vi "KE6221 -- Get Arb Wave Params.vi"(0 "Resource In":refnum<visa-resource-name>, 1 "Check For SCPI Errors? (T)":bool=TRUE, 11 "error in (no error)":errorcluster, 13 "Timeout (10000 ms)":u32=10000) -> (4 "Resource Out (dupl)":refnum<visa-resource-name>, 8 "Arb Wave Params":T1={"Frequency (Hz)"=1000.0, "Amplitude (A)"=0.001, "Offset (A)"=0.0, "Ranging Mode"=enum."Best", "Fixed Range"=enum."2mA", "Playback Mode"=enum."Time", "Time (s)"=1.0, "Num Cycles"=1.0, "Phase\nMarker?"=FALSE, "Phase Marker (deg)"=180.0, "Trig Link Line"=enum."1", "Arb Waveform Points"=[], "Num Arb Points"=0} {"Arb Waveform Points" min=-1.0 max=1.0 format="%.3f"; "Offset (A)" min=-0.105 max=0.105 format="%.4p"; "Num Cycles" min=0.001 max=99999999900.0 format="%.3p"; "Time (s)" min=1e-07 max=999999.999 format="%.3p"; "Phase Marker (deg)" min=0.0 max=360.0 format="%.3f"; "Amplitude (A)" min=2e-12 max=0.105 format="%.3p"; "Frequency (Hz)" min=0.001 max=100000.0 format="%.3p"}, 15 "error out":errorcluster)   [LabVIEW 2020, in "Keithley 622x.lvlib"]
doc: "Returns the parameters for the current arbitrary ('Arb') wave stored in location 0 (this is the non-volatile memory location), since this is the only location that can be read back remotely. Note that this VI can only be used with the 6221, since the 6220 doesn't support this feature."
uses:
  Keithley 622x.lvlib
  Low Level/Typedefs/KE6221 -- Wave Frequency.ctl
  Low Level/Typedefs/KE6221 -- Wave Amplitude.ctl
  Low Level/Typedefs/KE6221 -- Wave Ranging Mode.ctl
  Source/Typedefs/KE622x -- Current Ranges.ctl
  Low Level/Typedefs/KE6221 -- Wave Phase Marker.ctl
  Low Level/Typedefs/KE6221 -- Wave Playback Mode.ctl
  Low Level/Typedefs/KE6221 -- Wave Playback Time.ctl
  Low Level/Typedefs/KE6221 -- Wave Playback Num Cycles.ctl
  Source/Typedefs/KE622x -- Current Level.ctl
  Low Level/Typedefs/KE6221 -- Wave Arb Point.ctl
  Typedefs/KE6221 -- Wave Arb Wave Params.ctl
  C/Program Files/National Instruments/LabVIEW 2021/instr.lib/Keithley 622x LV 2009/Configure/Trigger/Low Level/Typedefs/KE622x -- Trig Link Line.ctl
panel:
  # "Note:  \"Arb Waveform Points\" and \"Num Arb Points\" refer to the Arb waveform in volatile memory (a.k.a. 'Location 0'). For the 'set' VI, the points are automatically copied into the specified non-volatile memory location."
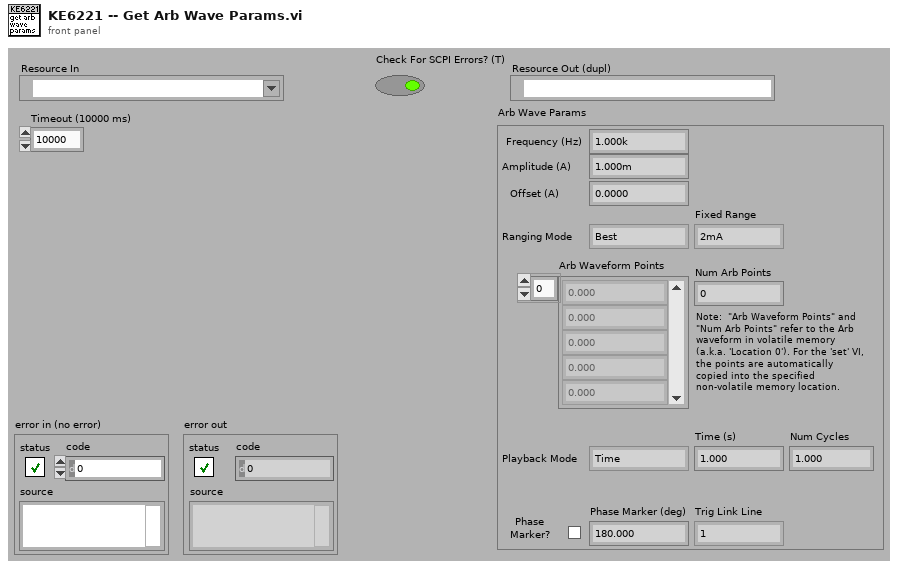
[diagram p1: front panel]
types:
  T1 = typedef "Keithley 622x.lvlib/KE6221 -- Wave Arb Wave Params.ctl" = cluster{"Frequency (Hz)":T2, "Amplitude (A)":T3, "Offset (A)":T4, "Ranging Mode":T5, "Fixed Range":T6, "Playback Mode":T7, "Time (s)":T8, "Num Cycles":T9, "Phase\nMarker?":bool, "Phase Marker (deg)":T10, "Trig Link Line":T11, "Arb Waveform Points":T12[], "Num Arb Points":u32}
  T2 = typedef "Keithley 622x.lvlib/KE6221 -- Wave Frequency.ctl" = dbl
  T3 = typedef "Keithley 622x.lvlib/KE6221 -- Wave Amplitude.ctl" = dbl
  T4 = typedef "Keithley 622x.lvlib/KE622x -- Current Level.ctl" = dbl
  T5 = typedef "Keithley 622x.lvlib/KE6221 -- Wave Ranging Mode.ctl" = enum16{"Best", "Fixed"}
  T6 = typedef "Keithley 622x.lvlib/KE622x -- Current Ranges.ctl" = enum16{"2nA", "20nA", "200nA", "2uA", "20uA", "200uA", "2mA", "20mA", "100mA"}
  T7 = typedef "Keithley 622x.lvlib/KE6221 -- Wave Playback Mode.ctl" = enum16{"Time", "Num Cycles"}
  T8 = typedef "Keithley 622x.lvlib/KE6221 -- Wave Playback Time.ctl" = dbl
  T9 = typedef "Keithley 622x.lvlib/KE6221 -- Wave Playback Num Cycles.ctl" = dbl
  T10 = typedef "Keithley 622x.lvlib/KE6221 -- Wave Phase Marker.ctl" = dbl
  T11 = typedef "Keithley 622x.lvlib/KE622x -- Trig Link Line.ctl" = enum16{"1", "2", "3", "4", "5", "6"}
  T12 = typedef "Keithley 622x.lvlib/KE6221 -- Wave Arb Point.ctl" = dbl
  T13 = typedef "Keithley 622x.lvlib/KE622x -- Current Range.ctl" = cluster{"Auto Range?":bool, "Man / Selected\nRange":T6}
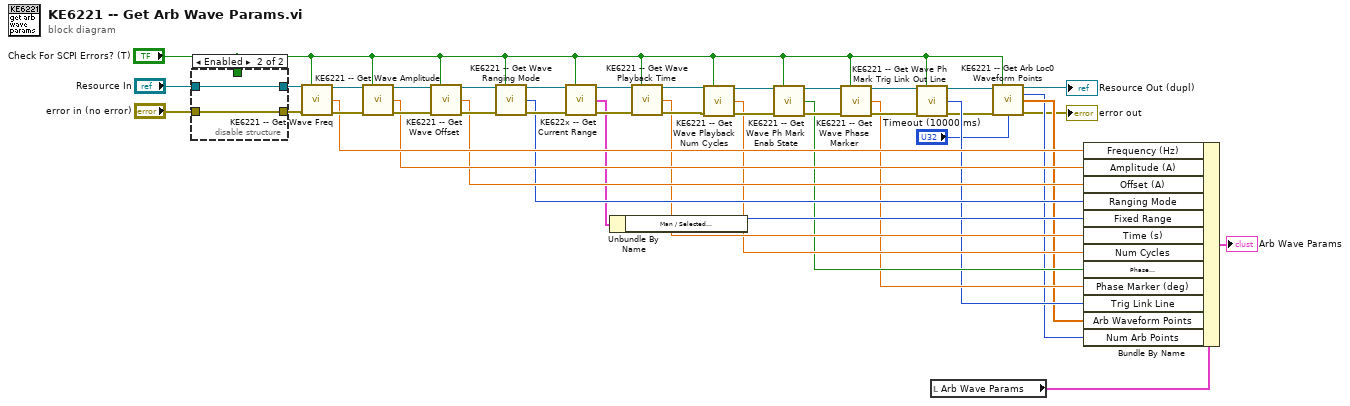
[diagram p0: block diagram]
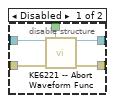
[diagram p2: hidden frame]
diagram:
  n1 = disable-structure shown="Enabled" {
    disable-tunnel: "Resource In" -> [w48 w50]
    disable-tunnel: "error in (no error)" -> [w47 w49]
    disable-tunnel: [w46 w49] -> w3
    disable-tunnel: [w45 w50] -> w2
    disable-tunnel: "Check For SCPI Errors? (T)" -> [w44 _]
    frame Disabled {
      n2 = call "KE6221 -- Abort Waveform Func.vi"("Resource In"=w48, "Check For SCPI Errors? (T)"=w44, "error in (no error)"=w47) -> ("Resource Out (dupl)"=w45:refnum<visa-resource-name>, "error out"=w46:errorcluster)  [unwired: 11 in]
    }
    frame Enabled {
    }
  }
  n3 = call "KE6221 -- Get Wave Freq.vi"("Resource In"=w2, "Check For SCPI Errors? (T)"="Check For SCPI Errors? (T)", "error in (no error)"=w3) -> ("Resource Out (dupl)"=w43:refnum<visa-resource-name>, "KE6221 Wave Freq (Hz)"=w24:T2, "error out"=w42:errorcluster)  [unwired: 10 in]
  n4 = call "KE6221 -- Get Wave Amplitude.vi"("Resource In"=w43, "Check For SCPI Errors? (T)"="Check For SCPI Errors? (T)", "error in (no error)"=w42) -> ("Resource Out (dupl)"=w39:refnum<visa-resource-name>, "Wave Amplitude"=w23:T3, "error out"=w38:errorcluster)  [unwired: 10 in]
  n5 = call "KE6221 -- Get Wave Offset.vi"("Resource In"=w39, "Check For SCPI Errors? (T)"="Check For SCPI Errors? (T)", "error in (no error)"=w38) -> ("Resource Out (dupl)"=w37:refnum<visa-resource-name>, "Wave Offset (A)"=w22:T4, "error out"=w36:errorcluster)  [unwired: 10 in]
  n6 = call "KE6221 -- Get Wave Ranging Mode.vi"("Resource In"=w37, "Check For SCPI Errors? (T)"="Check For SCPI Errors? (T)", "error in (no error)"=w36) -> ("Resource Out (dupl)"=w41:refnum<visa-resource-name>, "Ranging Mode"=w21:T5, "error out"=w40:errorcluster)  [unwired: 10 in]
  n7 = call "KE622x -- Get Current Range.vi"("Resource In"=w41, "Check For SCPI Errors? (T)"="Check For SCPI Errors? (T)", "error in (no error)"=w40) -> ("Resource Out (dupl)"=w35:refnum<visa-resource-name>, "Current Range"=w20:T13, "error out"=w34:errorcluster)  [unwired: 10 in]
  n8 = Unbundle By Name(w20) -> ("Man / Selected\nRange"=w19:T6)
  n9 = call "KE6221 -- Get Wave Playback Time.vi"("Resource In"=w35, "Check For SCPI Errors? (T)"="Check For SCPI Errors? (T)", "error in (no error)"=w34) -> ("Resource Out (dupl)"=w33:refnum<visa-resource-name>, "Playback Time (s)"=w18:T8, "error out"=w32:errorcluster)  [unwired: 10 in]
  n10 = call "KE6221 -- Get Wave Playback Num Cycles.vi"("Resource In"=w33, "Check For SCPI Errors? (T)"="Check For SCPI Errors? (T)", "error in (no error)"=w32) -> ("Resource Out (dupl)"=w31:refnum<visa-resource-name>, "Num Cycles"=w17:T9, "error out"=w30:errorcluster)  [unwired: 10 in]
  n11 = call "KE6221 -- Get Wave Ph Mark Enab State.vi"("Resource In"=w31, "Check For SCPI Errors? (T)"="Check For SCPI Errors? (T)", "error in (no error)"=w30) -> ("Resource Out (dupl)"=w29:refnum<visa-resource-name>, "Phase Marker Enabled?"=w16:bool, "error out"=w28:errorcluster)  [unwired: 10 in]
  n12 = call "KE6221 -- Get Wave Phase Marker.vi"("Resource In"=w29, "Check For SCPI Errors? (T)"="Check For SCPI Errors? (T)", "error in (no error)"=w28) -> ("Resource Out (dupl)"=w27:refnum<visa-resource-name>, "Phase Marker (deg)"=w15:T10, "error out"=w26:errorcluster)  [unwired: 10 in]
  n13 = call "KE6221 -- Get Wave Ph Mark Trig Link Out Line.vi"("Resource In"=w27, "Check For SCPI Errors? (T)"="Check For SCPI Errors? (T)", "error in (no error)"=w26) -> ("Resource Out (dupl)"=w13:refnum<visa-resource-name>, "Trig Link Out Line"=w14:T11, "error out"=w11:errorcluster)  [unwired: 10 in]
  n14 = local read "Arb Wave Params"() -> (w25:T1)
  n15 = call "KE6221 -- Get Arb Loc0 Waveform Points.vi"("Resource In"=w13, "Check For SCPI Errors? (T)"="Check For SCPI Errors? (T)", "error in (no error)"=w11, "Timeout (10000 ms)"="Timeout (10000 ms)") -> ("Resource Out (dupl)"=→"Resource Out (dupl)":refnum<visa-resource-name>, "Num Points"=w8:u32, "Arb Waveform Points"=w9:T12[], "error out"=→"error out":errorcluster)  [unwired: 8 in]
  n16 = Bundle By Name(cluster=w25, "Frequency (Hz)"=w24, "Amplitude (A)"=w23, "Offset (A)"=w22, "Ranging Mode"=w21, "Fixed Range"=w19, "Time (s)"=w18, "Num Cycles"=w17, "Phase\nMarker?"=w16, "Phase Marker (deg)"=w15, "Trig Link Line"=w14, "Arb Waveform Points"=w9, "Num Arb Points"=w8) -> (→"Arb Wave Params":T1)
